vi "Get Tag Settings.vi"(7 "Database Connection":refnum<k7>, 8 "Error In":errorcluster, 11 "TagId":string) -> (0 "Error Out":errorcluster, 3 "TagData":T1 {"Vmax" min=-10.0 max=10.0 step=1.0; "Vmin" min=-10.0 max=10.0 step=1.0})   [LabVIEW 2019]
uses:
  Controls/Tag Settings.ctl
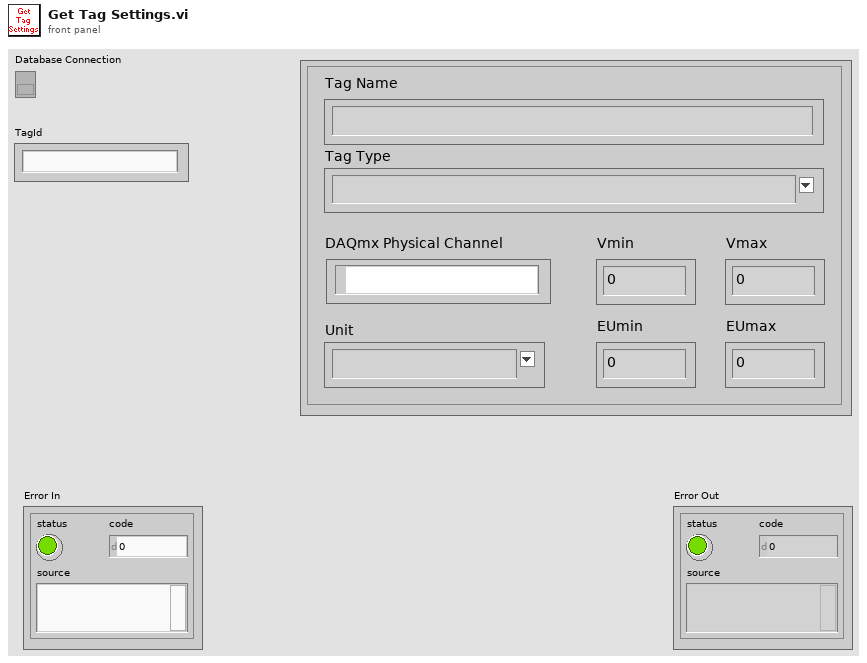
[diagram p1: front panel]
types:
  T1 = typedef "Tag Settings.ctl" = cluster{"Tag Name":string, "Tag Type":string, "DAQmx Physical Channel":tag, "Vmin":dbl, "Vmax":dbl, "Unit":string, "EUmin":dbl, "EUmax":dbl}
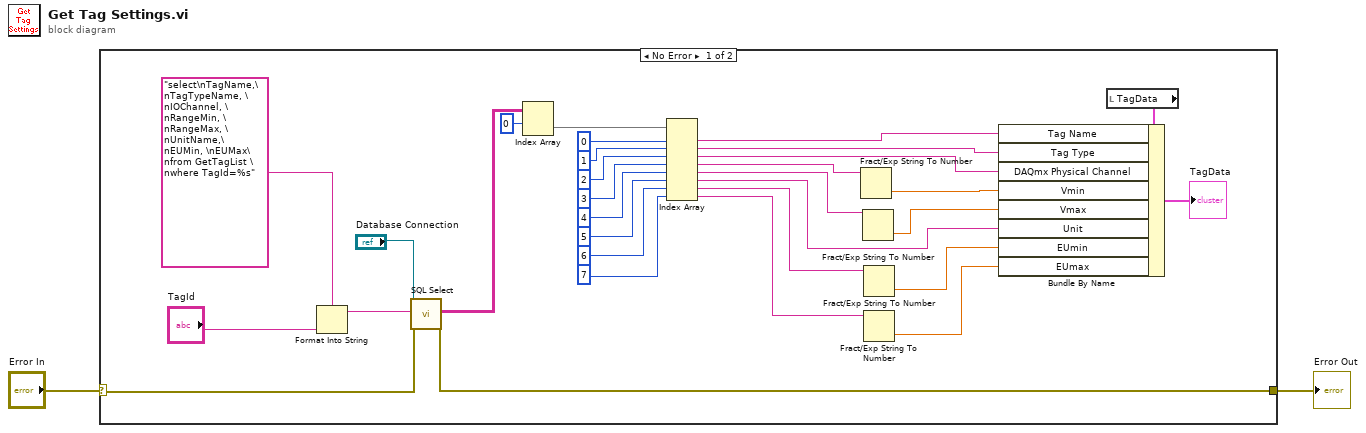
[diagram p0: block diagram]
diagram:
  n1 = case shown="No Error" "Error In" {
    selector: "Error In" -> [w32 w34]
    tunnel: [w31 w34] -> w1
    frame No Error {
      n2 = Format Into String(format string="select\nTagName,\nTagTypeName, \nIOChannel, \nRangeMin, \nRangeMax, \nUnitName,\nEUMin, \nEUMax\nfrom GetTagList \nwhere TagId=%s", "TagId") -> (resulting string=w28:string)  [unwired: 2 in, 1 out]
      n3 = call <vilib>:"SQL Select.vi"("Connection In"="Database Connection", "SQL Query"=w28, "Error in (no error)"=w32) -> ("Data"=w27:string[][], "Error out"=w31:errorcluster)  [unwired: 14 in, 1 out]
      n4 = Index Array "Index Array"(array=w27, index (row)=0) -> (element=w23:string[])  [unwired: 1 in]
      n5 = Index Array "Index Array"(array=w23, index #1=0 ("index"), index #2=1 ("index"), index #3=2 ("index"), index #4=3 ("index"), index #5=4 ("index"), index #6=5 ("index"), index #7=6 ("index"), index #8=7 ("index")) -> (element #1=w14:string, element #2=w13:string, element #3=w12:string, element #4=w11:string, element #5=w9:string, element #6=w7:string, element #7=w6:string, element #8=w4:string)
      n6 = Fract/Exp String To Number(string=w11) -> (number=w10:dbl)  [unwired: 3 in, 1 out]
      n7 = Fract/Exp String To Number(string=w9) -> (number=w8:dbl)  [unwired: 3 in, 1 out]
      n8 = Fract/Exp String To Number(string=w6) -> (number=w5:dbl)  [unwired: 3 in, 1 out]
      n9 = Fract/Exp String To Number(string=w4) -> (number=w3:dbl)  [unwired: 3 in, 1 out]
      n10 = local read "TagData"() -> (w25:T1)
      n11 = Bundle By Name(cluster=w25, "Tag Name"=w14, "Tag Type"=w13, "DAQmx Physical Channel"=w12, "Vmin"=w10, "Vmax"=w8, "Unit"=w7, "EUmin"=w5, "EUmax"=w3) -> (→"TagData":T1)
    }
    frame Error {
    }
  }
  "Error Out" <- w1
